vi "update.vi"(8 "error in (no error)":errorcluster, 11 "FPGAWrapperMH120124RAPS_PXI7813R in":refnum<class "FPGAWrapperMH120124RAPS_PXI7813R.lvclass">) -> (0 "error out":errorcluster, 3 "FPGAWrapperMH120124RAPS_PXI7813R out":refnum<class "FPGAWrapperMH120124RAPS_PXI7813R.lvclass">)   [LabVIEW 2010, in "FPGAWrapperMH120124RAPS_PXI7813R.lvclass"]
uses:
  FPGAWrapperMH120124RAPS_PXI7813R.lvclass
  grabber/command_enum.ctl
  FPGAWrapperMH120124RAPS_PXI7813R.lvclass/FPGAWrapperMH120124RAPS_PXI7813R.ctl
  class_data.vi
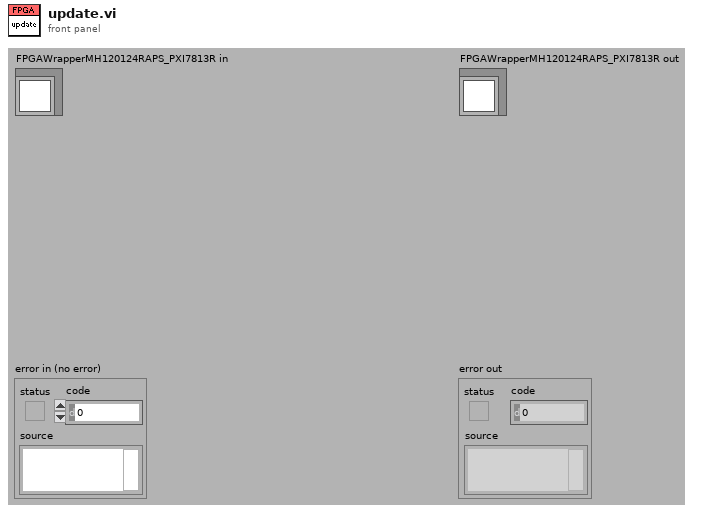
[diagram p1: front panel]
types:
  T1 = typedef "command_enum.ctl" = enum8{"NULL", "update", "start", "stop", "reset", "shut-down"}
  T2 = typedef "settings_cluster_raps.ctl" = cluster{"number of pixels":i32, "iterations per pixel":i32, "iterations per subpixel":i32, "maximum bit-depth":i8, "AOD center freq. (Hz)":dbl, "AOD bandwidth freq. (Hz)":dbl, "AOD amplitude":u16, "pixel dwell time":dbl, "AOD equilibration time":dbl, "ra trajectory pixels (data/pixels transfered)":u32, "pattern type":i8, "ellipsoid parameter cluster":T3, "pixel values cluster":T4, "offset (Hz)":dbl[], "RAPS array":u64[], "DDS board initialization parameters":T5, "gates":T6[]}
  T3 = typedef "ellipsoid_parameters_cluster.ctl" = cluster{"a":fxp<+/-,16,1>, "b":fxp<+/-,16,1>, "c":fxp<+/-,16,1>, "d":fxp<+/-,16,1>, "e":fxp<+/-,24,16>, "k":u16, "width":fxp<+,16,16>}
  T4 = typedef "channels_cluster.ctl" = cluster{"channel 0":u32, "channel 1":u32, "channel 2":u32, "channel 3":u32}
  T5 = typedef "DDS_board_init_cluster.ctl" = cluster{"Bypass PLL":bool, "PLL Range":bool, "Update Clock":bool, "Triangle ":bool, "SDO Active":bool, "LSB First":bool, "OSK Int":bool, "Output Shaped Keying Enable":bool, "Bypass Sinc":bool, "Digital Part":bool, "OutPut DAC":bool, "Control DAC":bool, "Comparator":bool, "Modus":u8, "Multiplier Value":u8}
  T6 = typedef "gate_cluster.ctl" = cluster{"index":i32, "parameters":T7}
  T7 = typedef "gate_parameters_cluster.ctl" = cluster{"offset":i64, "pulsing":i64, "not pulsing":i64, "cycles per pulse":i64, "repetitions":i64}
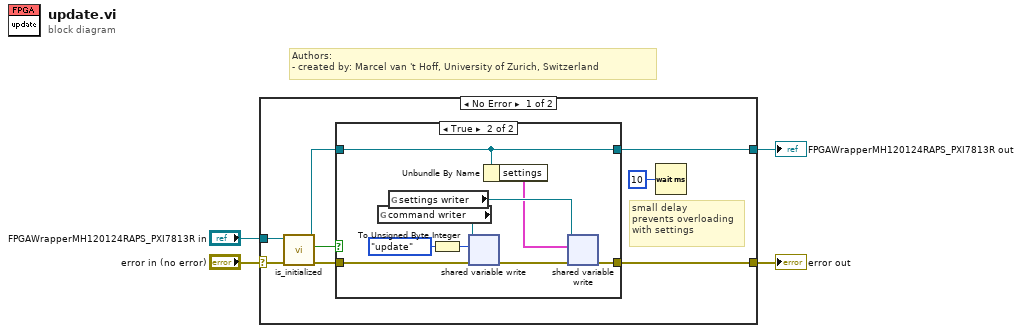
[diagram p0: block diagram]
diagram:
  # "Authors: \n- created by: Marcel van 't Hoff, University of Zurich, Switzerland"
  n1 = case shown="No Error" "error in (no error)" {
    selector: "error in (no error)" -> [w11 w25]
    tunnel: [w6 w25] -> w3
    tunnel: [w8 w24] -> w1
    tunnel: "FPGAWrapperMH120124RAPS_PXI7813R in" -> [w12 w24]
    frame No Error {
      # "small delay\nprevents overloading\nwith settings"
      n2 = call-dynamic "is_initialized.vi"("error in (no error)"=w11, "FPGAWrapperMH120124RAPS_PXI7813R in"=w12) -> ("error out"=w7:errorcluster, "is initialized?"=w10:bool, "FPGAWrapperMH120124RAPS_PXI7813R out"=w9:refnum<class "FPGAWrapperMH120124RAPS_PXI7813R.lvclass">)  [unwired: 7 in]
      n3 = case shown="True" w10 {
        tunnel: [w13 w20] -> w6
        tunnel: w9 -> [w14 w18]
        tunnel: w7 -> [w13 w19]
        tunnel: [w14 w18] -> w8
        frame False {
        }
        frame True {
          n4 = global read "class_data.vi" "command writer"() -> (w17:refnum<k21>)
          n5 = global read "class_data.vi" "settings writer"() -> (w16:refnum<k21>)
          n6 = To Unsigned Byte Integer(number=command_enum."update" ("command")) -> (unsigned 8bit integer=w23:u8)
          n7 = shared-variable-write(w17, w19, w23) -> (w21:errorcluster)  [unwired: 1 in, 2 out]
          n8 = Unbundle By Name(w18) -> ("settings"=w15:T2)
          n9 = shared-variable-write(w16, w21, w15) -> (w20:errorcluster)  [unwired: 1 in, 2 out]
        }
      }
      n10 = Wait (ms)(milliseconds to wait=u32 10) -> ()  [unwired: 1 out]
    }
    frame Error {
    }
  }
  "error out" <- w3
  "FPGAWrapperMH120124RAPS_PXI7813R out" <- w1
